vi "ROI entry screen-Adjust ROI Z values.vi"(9 "Old ROI file path":path, 10 "Old ROI file's data in":dbl[][](array[numeric]) format="%#_6f", 11 "ROI fit info":T1 {"ROI fit info"."Frame size"."Old" items=["100X100"=100, "128X128"=128, "200X200"=200, "256X256"=256, "512X512"=512, "1024x1024"=1024, "2048x2048"=2048]; "ROI fit info"."Frame size"."New" items=["100X100"=100, "128X128"=128, "200X200"=200, "256X256"=256, "512X512"=512, "1024x1024"=1024, "2048x2048"=2048]}) -> (1 "A Z coordinate could not be mapped":bool, 2 "Fitted ROI data":dbl[][](array[numeric]) format="%#_6f", 3 "Latest AOL Z (um)":dbl[](array[numeric]))   [LabVIEW 2013]
uses:
  Typedefs/ROI fitting info cluster.ctl
  Typedefs/Frame Size.ctl
panel:
  # "X start"
  # "Y start"
  # "Z start"
  # "X stop"
  # "Y stop"
  # "Z stop"
  # "X start"
  # "Y start"
  # "Z start"
  # "X stop"
  # "Y stop"
  # "Z stop"
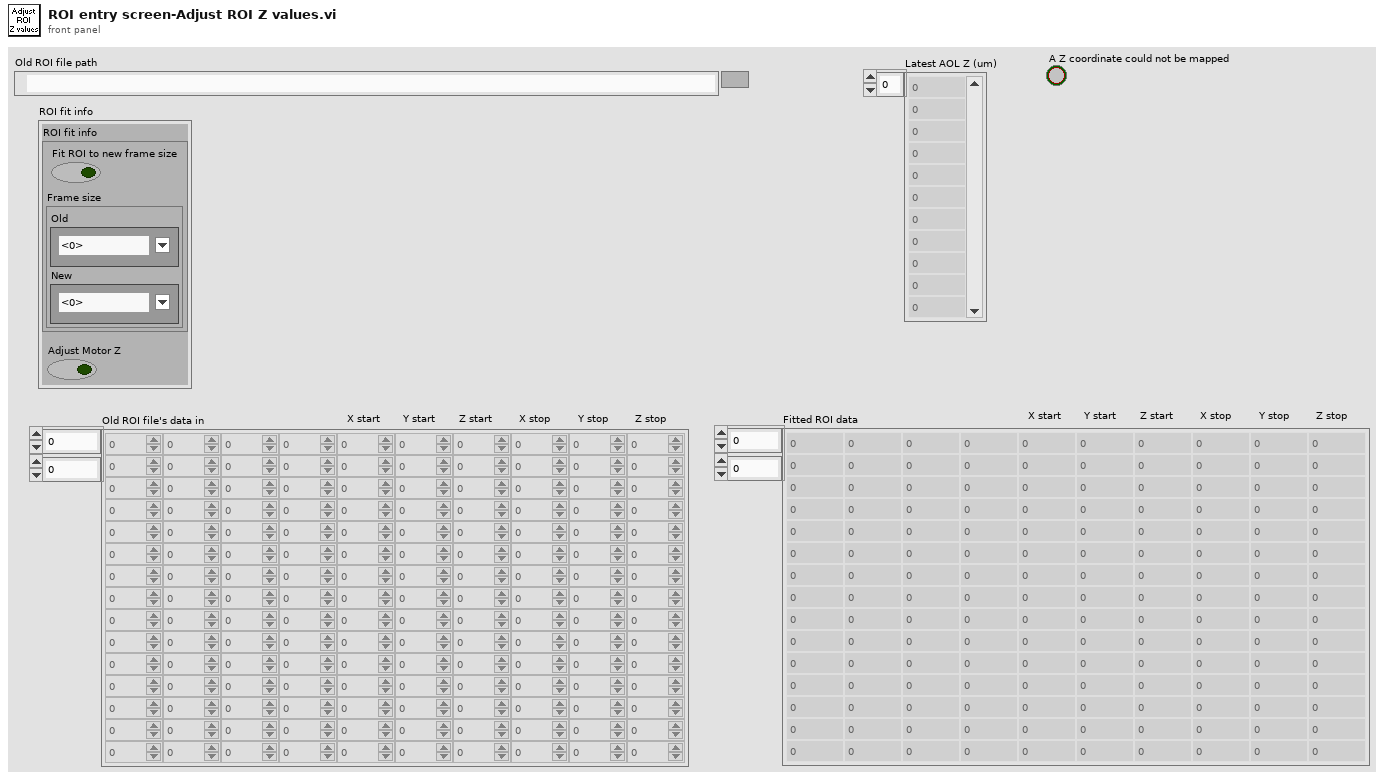
[diagram p1: front panel]
types:
  T1 = typedef "ROI fitting info cluster.ctl" = cluster{"ROI fit info":cluster{"Fit ROI to new frame size":bool, "Frame size":cluster{"Old":T2, "New":T2}}, "Adjust Motor Z":bool}
  T2 = typedef "Frame Size.ctl" = u16
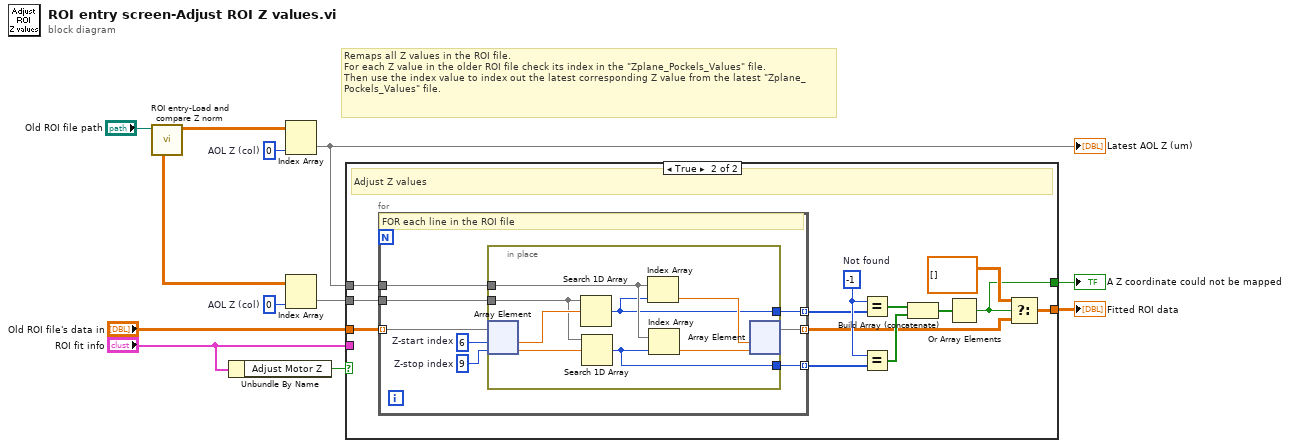
[diagram p0: block diagram]
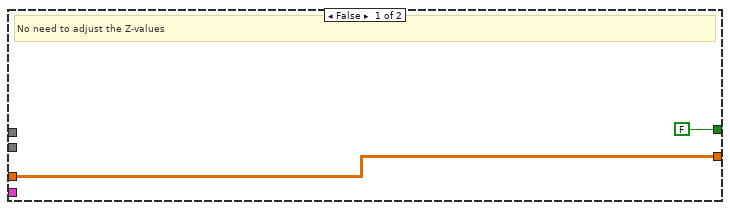
[diagram p2: hidden frame]
diagram:
  w6 = 0  # AOL Z (col)
  w8 = 0  # AOL Z (col)
  # "Remaps all Z values in the ROI file.\nFor each Z value in the older ROI file check its index in the \"Zplane_Pockels_Values\" file.\nThen use the index value to index out the latest corresponding Z value from the latest \"Zplane_Pockels_Values\" file."
  n1 = call "ROI entry-Load and compare Z norm.vi"("Old ROI file path"="Old ROI file path") -> ("Latest Zplane_Pockels_Values file data (header removed)"=w9:dbl[][], "Older Zplane_Pockels_Values file data (header removed)"=w5:dbl[][])  [unwired: 4 in, 5 out]
  n2 = Unbundle By Name("ROI fit info") -> ("Adjust Motor Z"=w12:bool)
  n3 = Index Array(array=w9, index (col)=w8) -> (element=w3:dbl[])  [unwired: 1 in]
  "Latest AOL Z (um)" <- w3
  n4 = Index Array(array=w5, index (col)=w6) -> (element=w4:dbl[])  [unwired: 1 in]
  n5 = case shown="True" w12 {
    tunnel: "Old ROI file's data in" -> [w14 w27]
    tunnel: "ROI fit info" -> [_ _]
    tunnel: w4 -> [_ w26]
    tunnel: w3 -> [_ w25]
    tunnel: [FALSE w19] -> w2
    tunnel: [w14 w15] -> w1
    frame False {
      # "No need to adjust the Z-values"
    }
    frame True {
      w20 = -1  # Not found
      # "Adjust Z values"
      n6 = for {
        tunnel: w27 -> [w35] mode=indexing
        tunnel: [w32] -> w18 mode=indexing
        tunnel: w26 -> [w31]
        tunnel: w25 -> [w30]
        tunnel: [w29] -> w17 mode=indexing
        tunnel: [w28] -> w16 mode=indexing
        w33 = 9  # Z-stop index
        w34 = 6  # Z-start index
        # "FOR each line in the ROI file"
        n7 = in-place {
          in-place-border: w31 -> [w39]
          in-place-border: w30 -> [w40]
          in-place-border: [w37] -> w29
          in-place-border: [w36] -> w28
          n8 = in-place-array #1(w35, w34, w33) -> (w43:dbl, w38:dbl)
          n9 = Search 1D Array(1D array=w39, element=w43) -> (index of element=w37:i32)  [unwired: 1 in]
          n10 = Search 1D Array(1D array=w39, element=w38) -> (index of element=w36:i32)  [unwired: 1 in]
          n11 = Index Array(array=w40, index=w37) -> (element=w42:dbl)
          n12 = Index Array(array=w40, index=w36) -> (element=w41:dbl)
          n13 = in-place-array #1(w42, w41) -> (w32:dbl[])  [unwired: 2 out]
        }
      }
      n14 = Equal?(x=w20, y=w17) -> (x = y?=w21:bool[])
      n15 = Equal?(x=w20, y=w16) -> (x = y?=w22:bool[])
      n16 = Build Array (concatenate)(w21, w22) -> (w23:bool[])
      n17 = Or Array Elements(Boolean array=w23) -> (logical OR=w19:bool)
      n18 = Select(t=dbl[][] [], s=w19, f=w18) -> (s? t:f=w15:dbl[][])
    }
  }
  "Fitted ROI data" <- w1
  "A Z coordinate could not be mapped" <- w2
